vi "TDMS Export Data Events.vi"(6 "Time Stamps":cluster{"Start":timestamp, "End":timestamp}, 8 "error in (no error)":errorcluster, 9 "Output Directory":path, 10 "Asset":string, 11 "InsightCM Console Wrapper in":refnum<class "InsightCM Console Wrapper.lvclass">) -> (0 "error out":errorcluster, 3 "InsightCM Console Wrapper out":refnum<class "InsightCM Console Wrapper.lvclass">)   [LabVIEW 2020, in "InsightCM Console Wrapper.lvclass"]
doc: "Exports datasets as a TDMS File.\n\nConsole commands\n\n-> exporttdms -id [data event id] -o [filepath] - [Not implemented yet]\n-> exporttdms -dir [directory] -asset [asset path] -start [start date yyyy-mm-dd] -end [end date yyyy-mm-dd])"
uses:
  InsightCM Console Wrapper.lvclass
  C:/Users/fflores/Documents/GitHub Projects/LabVIEW-CLI-Wrapper/Console Wrapper/Console Wrapper.lvclass
  Console Wrapper/Console Wrapper.lvclass/Console Wrapper.ctl
  Console Wrapper/Write Command Options.vi
  Console Wrapper/Write Command.vi
  Console Wrapper/Console Wrapper.lvclass
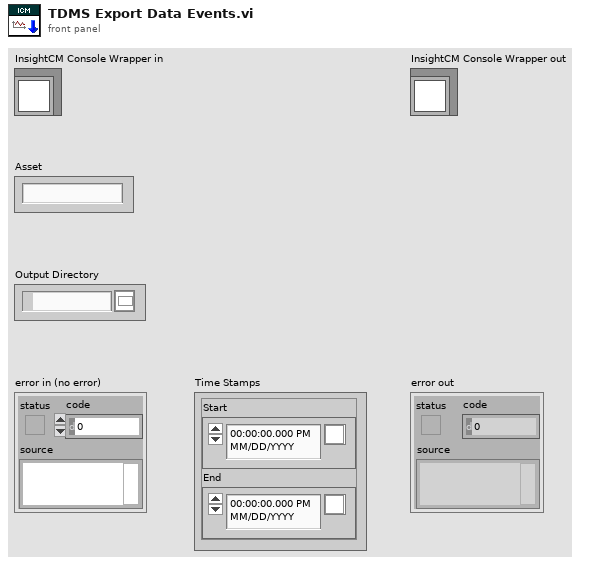
[diagram p1: front panel]
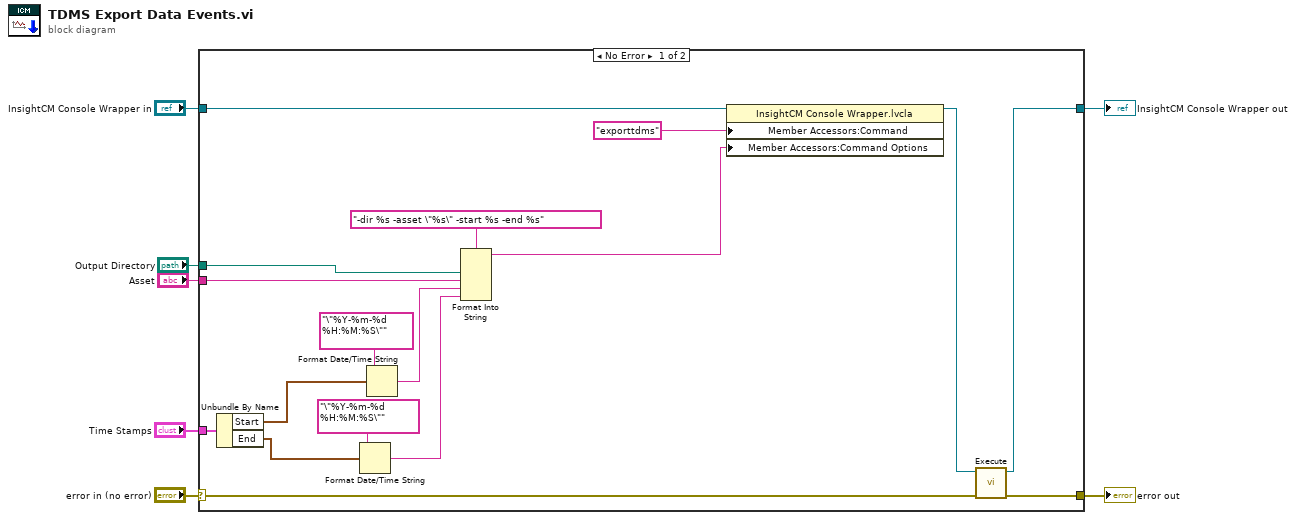
[diagram p0: block diagram]
diagram:
  n1 = case shown="No Error" "error in (no error)" {
    selector: "error in (no error)" -> [w24 w26]
    tunnel: [w23 w26] -> w6
    tunnel: [w21 w25] -> w4
    tunnel: "InsightCM Console Wrapper in" -> [w22 w25]
    tunnel: "Time Stamps" -> [w16 _]
    tunnel: "Asset" -> [w11 _]
    tunnel: "Output Directory" -> [w12 _]
    frame No Error {
      n2 = Unbundle By Name(w16) -> ("Start"=w15:timestamp, "End"=w14:timestamp)
      n3 = Format Date/Time String(time format string (%c)="\"%Y-%m-%d %H:%M:%S\"", seconds (now)=w14) -> (date/time string=w9:string)  [unwired: 1 in]
      n4 = Format Date/Time String(time format string (%c)="\"%Y-%m-%d %H:%M:%S\"", seconds (now)=w15) -> (date/time string=w10:string)  [unwired: 1 in]
      n5 = Format Into String(format string="-dir %s -asset \"%s\" -start %s -end %s", w12, w11, w10, w9) -> (resulting string=w8:string)  [unwired: 2 in, 1 out]
      n6 = property class="InsightCM Console Wrapper.lvcla"(reference=w22, "Member Accessors:Command"="exporttdms" ("Command"), "Member Accessors:Command Options"=w8) -> (reference out=w20:refnum<class "InsightCM Console Wrapper.lvclass">)  [unwired: 1 in, 1 out]
      n7 = call "Execute.vi"("error in (no error)"=w24, "Console Wrapper in"=w20) -> ("error out"=w23:errorcluster, "Console Wrapper out"=w21:refnum<class "InsightCM Console Wrapper.lvclass">)  [unwired: 7 in, 1 out]
    }
    frame Error {
    }
  }
  "error out" <- w6
  "InsightCM Console Wrapper out" <- w4
